vi "Generate User Event.vi"() -> ()   [LabVIEW 2024]
uses:
  User Events.lvlib
panel:
  in  "stop":bool
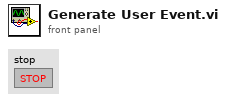
[diagram p1: front panel]
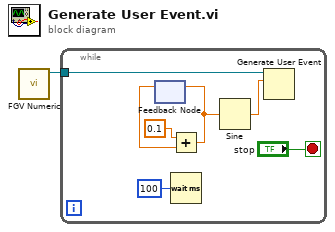
[diagram p0: block diagram]
diagram:
  n1 = call "FGV Numeric.vi"() -> ("Numeric UE"=w1:refnum<user-event>)  [unwired: 11 in]
  n2 = while {
    tunnel: w1 -> [w8]
    stop <- "stop" stop-if-true
    n3 = feedback #1() -> (w7:dbl)  [unwired: 1 in]
    n4 = Add(x=0.1, y=w7) -> (x+y=w5:dbl)
    n5 = feedback-in #1(w5) -> ()
    n6 = Wait (ms)(milliseconds to wait=u32 100) -> ()  [unwired: 1 out]
    n7 = Sine(x=w5) -> (sin(x)=w4:dbl)
    n8 = Generate User Event(user event=w8, event data cluster=w4) -> ()  [unwired: 2 in, 2 out]
  }
